vi "Clip AO Waveforms.vi"(8 "error in (no error)":errorcluster, 10 "AO []":waveform(dbl)[](array[waveform]), 11 "Instrument.DAQ in":refnum<class "Instrument.DAQ.lvclass">) -> (0 "error out":errorcluster, 2 "Clipped AO []":waveform(dbl)[](array[waveform]), 3 "Instrument.DAQ out":refnum<class "Instrument.DAQ.lvclass">)   [LabVIEW 2019, in "Instrument.DAQ.lvclass"]
uses:
  Instrument.DAQ.lvclass
  Instrument.DAQ.lvclass/Instrument.DAQ.ctl
  <resource>/objmgr/daqmx.rc
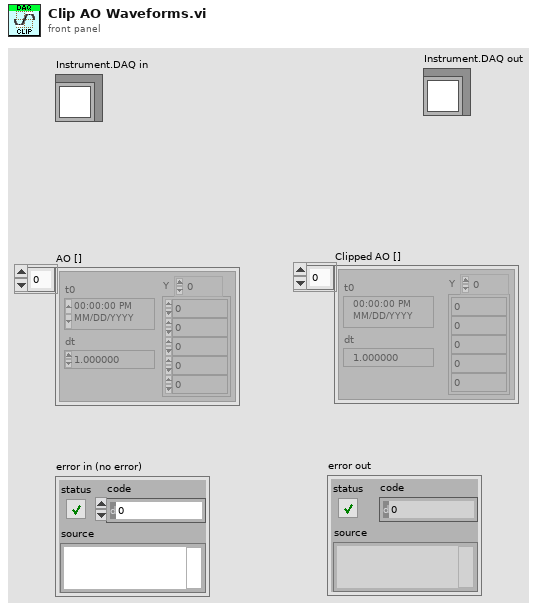
[diagram p1: front panel]
types:
  T1 = typedef "Instrument.DAQ.lvclass/DAQ.Config.AO--Cluster--Array.ctl" = T2[]
  T2 = typedef "Instrument.DAQ.lvclass/DAQ.Config.AO--Cluster.ctl" = cluster{"Channels":tag, "Range":T3, "output terminal configuration":i32, "Type":T4}
  T3 = typedef "Instrument.DAQ.lvclass/DAQ.Config.AO.Range--enum.ctl" = enum16{"±0.1", "±1.0", "±10.0"}
  T4 = typedef "Instrument.DAQ.lvclass/DAQ.Type--enum.ctl" = enum16{"None", "USB-4431", "PXI-446x"}
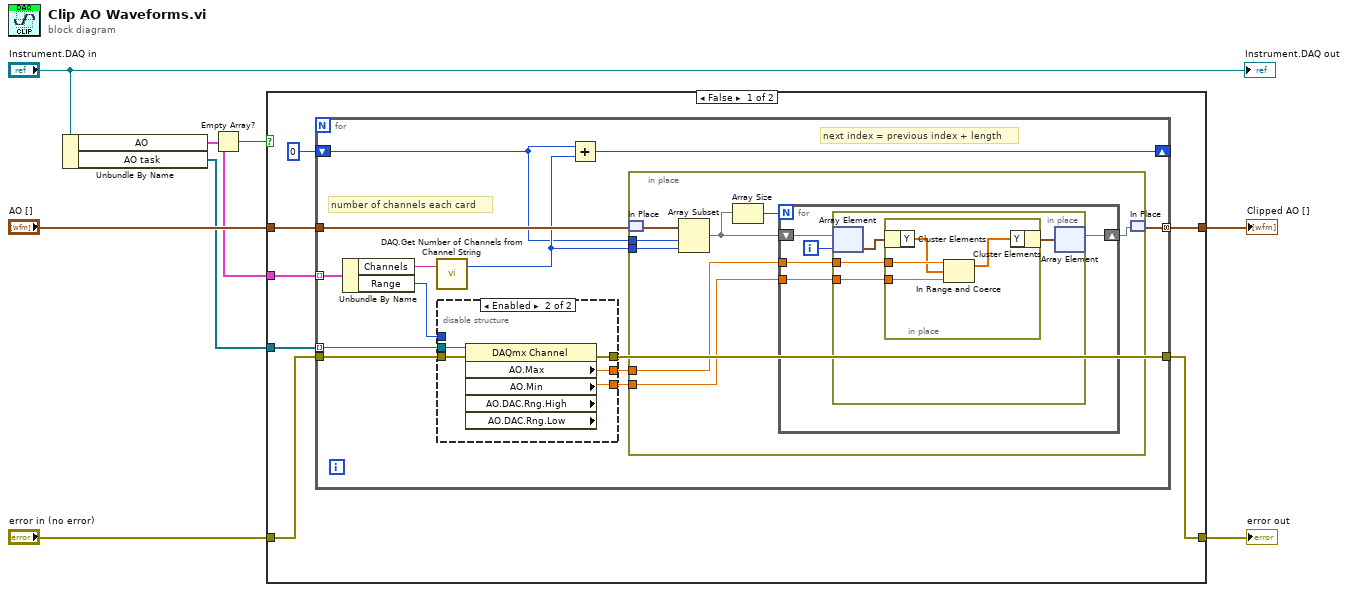
[diagram p0: block diagram]
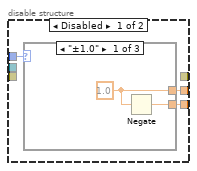
[diagram p2: hidden frame]
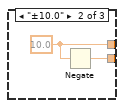
[diagram p3: hidden frame]
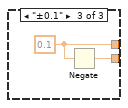
[diagram p4: hidden frame]
diagram:
  n1 = Unbundle By Name("Instrument.DAQ in") -> ("AO"=w4:T1, "AO task"=w3:refnum<k21>[])
  n2 = Empty Array?(array=w4) -> (empty?=w6:bool)
  n3 = case shown="False" w6 {
    tunnel: [w15 w65] -> w8
    tunnel: "AO []" -> [w14 w65]
    tunnel: w4 -> [w13 _]
    tunnel: w3 -> [w11 _]
    tunnel: "error in (no error)" -> [w10 w64]
    tunnel: [w9 w64] -> w1
    frame False {
      n4 = for {
        tunnel: w13 -> [w28] mode=indexing
        tunnel: w14 -> [w22]
        tunnel: [w23] -> w15 mode=concatenating
        shift-right: [w21] -> _
        shift-left: 0 -> [w19]
        tunnel: w11 -> [w18] mode=indexing
        tunnel: w10 -> [w17]
        tunnel: [w16] -> w9
        # "next index = previous index + length"
        # "number of channels each card"
        n5 = Unbundle By Name(w28) -> ("Channels"=w25:tag, "Range"=w24:T3)
        n6 = call "DAQ.Get Number of Channels from Channel String.vi"("Channels String"=w25) -> ("# channels"=w20:i32)  [unwired: 2 in]
        n7 = disable-structure shown="Enabled" {
          disable-tunnel: [w31 w42] -> w27
          disable-tunnel: [w30 w41] -> w26
          disable-tunnel: w24 -> [w29 _]
          disable-tunnel: w18 -> [_ w40]
          disable-tunnel: w17 -> [_ w39]
          disable-tunnel: [_ w38] -> w16
          frame Disabled {
            n8 = case shown="\"±1.0\"" w29 {
              tunnel: [w33 w35 w37] -> w31
              tunnel: [w32 w34 w36] -> w30
              frame "±1.0" {
                w33 = 1.0
                n9 = Negate(x=w33) -> (-x=w32:dbl)
              }
              frame "±10.0" {
                w35 = 10.0
                n10 = Negate(x=w35) -> (-x=w34:dbl)
              }
              frame "±0.1" {
                w37 = 0.1
                n11 = Negate(x=w37) -> (-x=w36:dbl)
              }
            }
          }
          frame Enabled {
            n12 = property class="DAQmx Channel" props=["AO.Max", "AO.Min", "AO.DAC.Rng.High", "AO.DAC.Rng.Low"](reference=w40, error in=w39) -> (error out=w38:errorcluster, "AO.Max"=w42:dbl, "AO.Min"=w41:dbl)  [unwired: 3 out]
          }
        }
        n13 = Add(x=w19, y=w20) -> (x+y=w21:i32)
        n14 = in-place {
          in-place-border: w20 -> [w50]
          in-place-border: w19 -> [w49]
          in-place-border: w27 -> [w48]
          in-place-border: w26 -> [w47]
          n15 = in-place-match #1(w22) -> (w46:waveform(dbl)[])
          n16 = Array Subset(array=w46, index=w49, length=w50) -> (w43:waveform(dbl)[])
          n17 = Array Size(array=w43) -> (size(s)=w44:i32)
          n18 = for {
            N: w44 -> [_]
            tunnel: w48 -> [w55]
            tunnel: w47 -> [w54]
            shift-right: [w51] -> w45
            shift-left: w43 -> [w52]
            i -> [w53]
            n19 = in-place {
              in-place-border: w55 -> [w59]
              in-place-border: w54 -> [w58]
              n20 = in-place-array #2(w52, w53) -> (w57:waveform(dbl))
              n21 = in-place {
                in-place-border: w59 -> [w63]
                in-place-border: w58 -> [w62]
                n22 = in-place-cluster #3(w57) -> ("Y"=w61:dbl[])
                n23 = In Range and Coerce(upper limit=w63, x=w61, lower limit=w62) -> (coerced(x)=w60:dbl[])  [unwired: 1 out]
                n24 = in-place-cluster #3("Y"=w60) -> (w56:waveform(dbl))
              }
              n25 = in-place-array #2(w56) -> (w51:waveform(dbl)[])  [unwired: 1 out]
            }
          }
          n26 = in-place-match #1(w45) -> (w23:waveform(dbl)[])
        }
      }
    }
    frame True {
      # "If AO Config = empty, do nothing"
    }
  }
  "Clipped AO []" <- w8
  "error out" <- w1
  "Instrument.DAQ out" <- "Instrument.DAQ in"
